vi "Image in Header or Footer.vi"(0 "report in":refnum<class "NI_report.lvclass">, 5 "select header or footer":u16(ring) items=["Left Header", "Left Footer", "Center Header", "Center Footer", "Right Herader", "Right Footer"], 9 "image path":string, 11 "error in (no error)":errorcluster, 12 "text above image":string) -> (4 "report out":refnum<class "NI_report.lvclass">, 15 "error out":errorcluster)   [LabVIEW 2020, in "NI_report.lvclass"]
doc: "This VI sets an image for the report header or footer.\n\nRemember, with the HTML report type the left, center, and right header texts are placed on separate lines."
uses:
  <vilib>/Utility/NIReport.llb/NI_report.lvclass
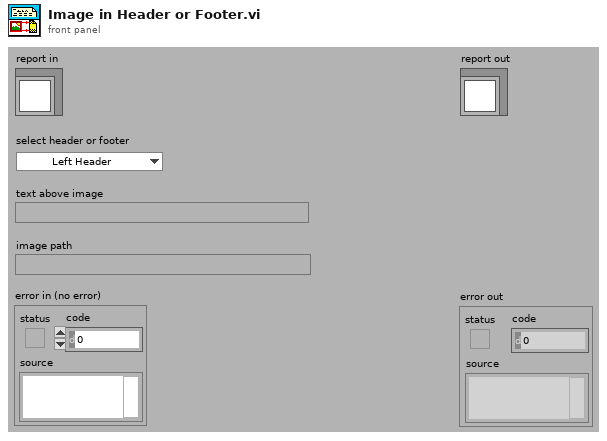
[diagram p1: front panel]
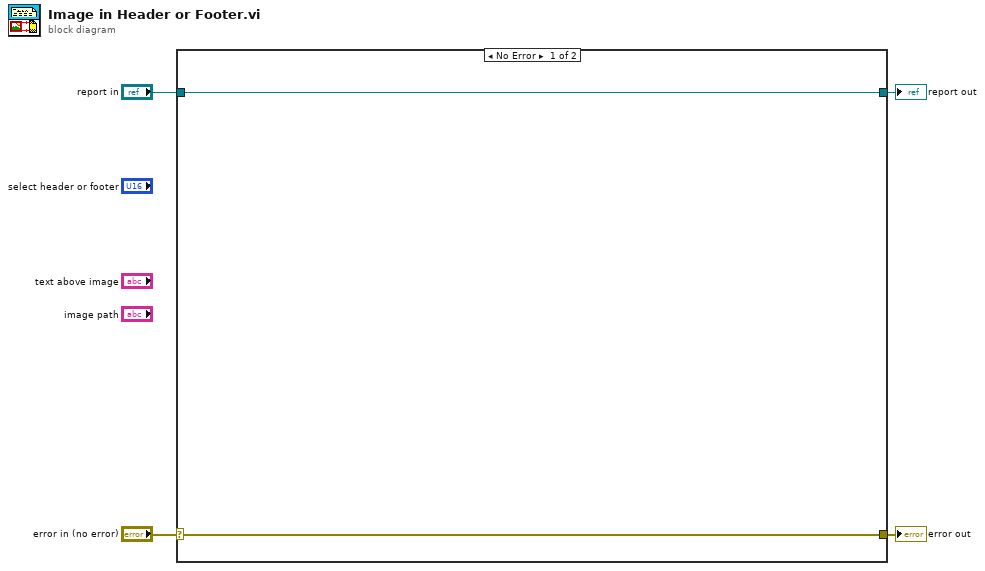
[diagram p0: block diagram]
diagram:
  n1 = case shown="No Error" "error in (no error)" {
    selector: "error in (no error)" -> [w6 w8]
    tunnel: [w6 w8] -> w3
    tunnel: [w5 w7] -> w1
    tunnel: "report in" -> [w5 w7]
    frame No Error {
    }
    frame Error {
    }
  }
  "error out" <- w3
  "report out" <- w1
